vi "Endpoint Connected.vi"(8 "error in (no error)":errorcluster, 10 "Endpoint Enqueuer":refnum<class "Message Enqueuer.lvclass">, 11 "Cobra RT in":refnum<class "Cobra RT.lvclass">) -> (0 "error out":errorcluster, 3 "Cobra RT out":refnum<class "Cobra RT.lvclass">)   [LabVIEW 2019, in "Cobra RT.lvlib" / "Cobra RT.lvclass"]
uses:
  Cobra RT.lvclass
  <vilib>/ActorFramework/Message Enqueuer/Message Enqueuer.lvclass
  Cobra RT.lvclass/Cobra RT.ctl
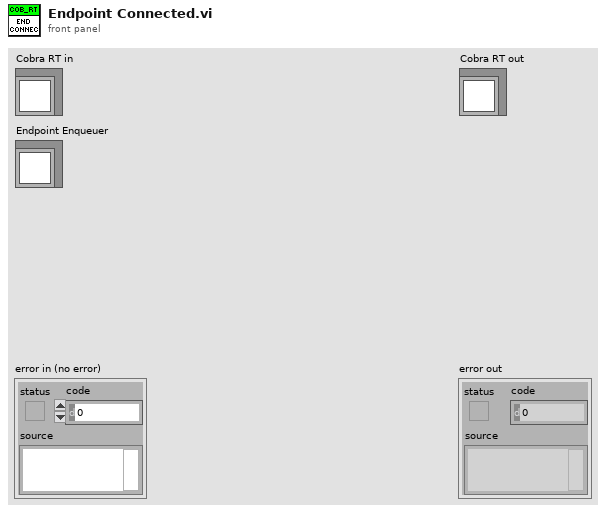
[diagram p1: front panel]
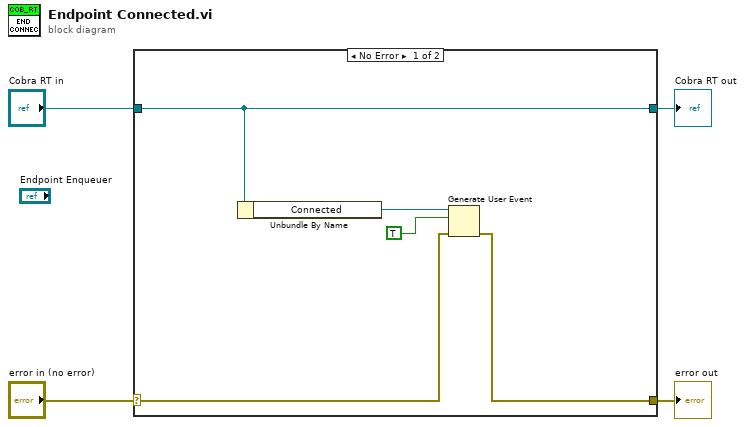
[diagram p0: block diagram]
diagram:
  n1 = case shown="No Error" "error in (no error)" {
    selector: "error in (no error)" -> [w5 w11]
    tunnel: [w9 w11] -> w3
    tunnel: [w6 w10] -> w1
    tunnel: "Cobra RT in" -> [w6 w10]
    frame No Error {
      n2 = Unbundle By Name(w6) -> ("Connected"=w7:refnum<user-event>)
      n3 = Generate User Event(user event=w7, event data cluster=TRUE ("event data"), error in=w5) -> (error out=w9:errorcluster)  [unwired: 1 in, 1 out]
    }
    frame Error {
    }
  }
  "error out" <- w3
  "Cobra RT out" <- w1
